vi "Stop Core.vi"(10 "final error code":i32, 11 "Nested in":refnum<class "Object Dictionary UI.lvclass">) -> (3 "Nested out":refnum<class "Object Dictionary UI.lvclass">)   [LabVIEW 2024, in "Object Dictionary UI.lvlib" / "Object Dictionary UI.lvclass"]
doc: "(<B>Filename</B>: Actor Framework.lvlib:Actor.lvclass:Stop Core.vi)\n\nDefines what the actor does before it stops. Use the <B>final error code</B> input to determine whether the actor shut down in response to an error.\n\nBy default, this method does nothing. A descendant class may override it to define behavior, such as shutting down any processes the actor initiated in its override of the Actor Core method."
uses:
  Object Dictionary UI.lvclass
  <vilib>/MGI/Panel Manager/Panel Actor/Panel Actor/Panel Actor.lvclass
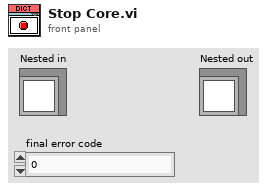
[diagram p1: front panel]
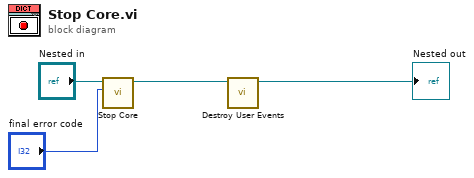
[diagram p0: block diagram]
diagram:
  n1 = call-parent "Stop Core.vi"("final error code"="final error code", "Actor in"="Nested in") -> ("Actor out"=w2:refnum<class "Object Dictionary UI.lvclass">)  [unwired: 9 in]
  n2 = call "Destroy User Events.vi"("UI Template in"=w2) -> ("UI Template out"=→"Nested out":refnum<class "Object Dictionary UI.lvclass">)  [unwired: 10 in]
